vi "Log Audit.vi"(8 "error in":errorcluster, 10 "Audit Event":refnum<class "Audit Event.lvclass">, 11 "Data":refnum<class "Logging Service.lvclass">) -> (0 "error out":errorcluster)   [LabVIEW 2026, in "Logging Service.lvclass"]
uses:
  Logging Service.lvclass
  Logging Service.lvclass/Logging Service.ctl
  Domain/Audit Event/Audit Event.lvclass
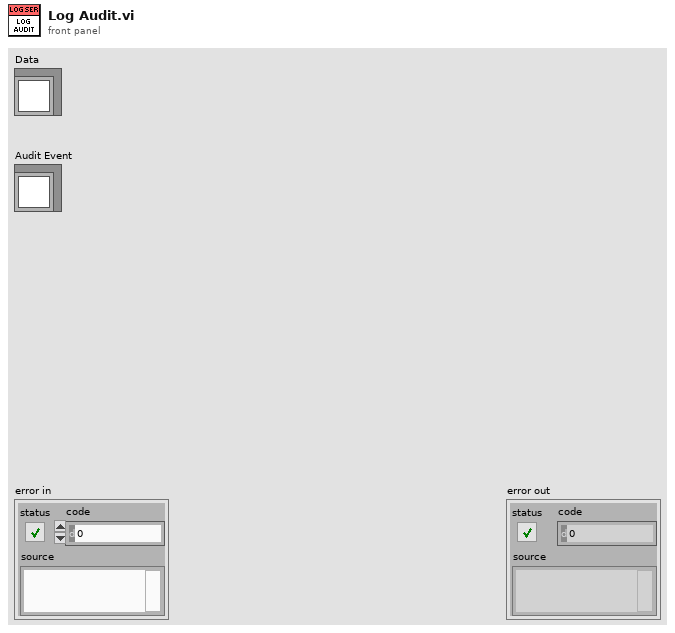
[diagram p1: front panel]
types:
  T1 = enum16{"open", "replace", "create", "open or create", "replace or create", "replace or create with confirmation"}
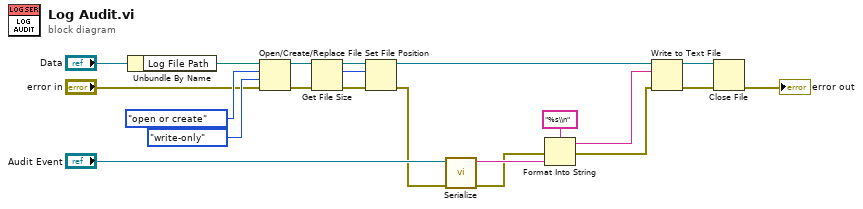
[diagram p0: block diagram]
diagram:
  n1 = Unbundle By Name("Data") -> ("Log File Path"=w20:path)
  n2 = Open/Create/Replace File(file path (use dialog)=w20, error in="error in", operation (0:open)=T1."open or create", access (0:read/write)=enum16{"read/write", "read-only", "write-only"}."write-only") -> (refnum out=w16:refnum<file>, error out=w15:errorcluster)  [unwired: 2 in, 1 out]
  n3 = Get File Size(file=w16, error in=w15) -> (refnum out=w14:refnum<file>, size (in bytes)=w12:i64, 0:w13:errorcluster)
  n4 = Set File Position(offset (in bytes) (0)=w12, refnum=w14, error in=w13) -> (refnum out=w11:refnum<file>, error out=w2:errorcluster)  [unwired: 1 in]
  n5 = call "Serialize.vi"("error in (no error)"=w2, "Audit Event"="Audit Event") -> ("error out"=w1:errorcluster, "Serialized Audit Event"=w3:string)  [unwired: 8 in]
  n6 = Format Into String(format string="%s\\n", error in=w1, w3) -> (resulting string=w5:string, error out=w6:errorcluster)  [unwired: 1 in]
  n7 = Write to Text File(file (use dialog)=w11, text=w5, error in=w6) -> (refnum out=w9:refnum<file>, error out=w10:errorcluster)  [unwired: 1 in, 1 out]
  n8 = Close File(refnum=w9, error in=w10) -> (error out=→"error out":errorcluster)  [unwired: 1 out]
